vi "Read Operator Joystick.vi"   [LabVIEW 2020]
uses:
  Framework/Robot Global Data.vi
  <vilib>/Rock Robotics/Network Tables/NT Write Numeric Array.vi
  <vilib>/Rock Robotics/Network Tables/NT Write Boolean Array.vi
types:
  T1 = enum16{"0", "1", "2", "3", "4", "5", "6", "7", "8", "9", "10", "11"}
  T2 = typedef "WPI_JoystickDevRef.ctl" = cluster{"Device":T3}
  T3 = typedef "WPI_JoystickDeviceEnum.ctl" = enum16{"USB 0", "USB 1", "USB 2", "USB 3", "USB 4", "USB 5"}
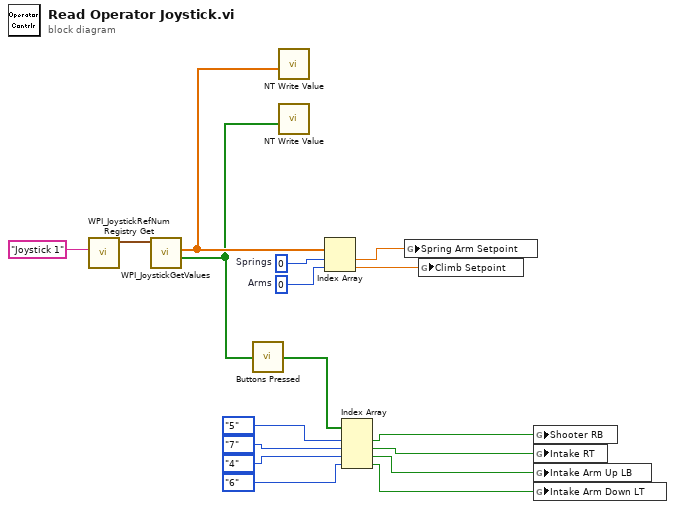
[diagram p0: block diagram]
diagram:
  w14 = 0  # Arms
  w15 = 0  # Springs
  n1 = call <vilib>:"WPI_JoystickRefNum Registry Get.vi"("refnum name"="Joystick 1") -> ("JoystickDevRef"=w17:T2)  [unwired: 9 in, 1 out]
  n2 = call <vilib>:"WPI_JoystickGetValues.vi"("JoystickDevRef"=w17) -> ("Buttons"=w12:bool[], "Axes"=w13:dbl[])  [unwired: 6 in, 3 out]
  n3 = call "Buttons Pressed.vi"("Button Values"=w12) -> ("Button Presses"=w11:bool[])
  n4 = call-poly <vilib>:"NT Write Value.vi"("Numeric Array"=w13) -> ()  [unwired: 10 in, 1 out]
  n5 = call-poly <vilib>:"NT Write Value.vi"("Boolean Array"=w12) -> ()  [unwired: 10 in, 1 out]
  n6 = Index Array(array=w13, index #1=w15, index #2=w14) -> (element #1=w10:dbl, element #2=w9:dbl)
  n7 = Index Array(array=w11, index #1=T1."5", index #2=T1."7", index #3=T1."4", index #4=T1."6") -> (element #1=w8:bool, element #2=w7:bool, element #3=w6:bool, element #4=w5:bool)
  n8 = global write "Robot Global Data.vi" "Spring Arm Setpoint"(w10) -> ()
  n9 = global write "Robot Global Data.vi" "Climb Setpoint"(w9) -> ()
  n10 = global write "Robot Global Data.vi" "Shooter RB"(w8) -> ()
  n11 = global write "Robot Global Data.vi" "Intake RT"(w7) -> ()
  n12 = global write "Robot Global Data.vi" "Intake Arm Up LB"(w6) -> ()
  n13 = global write "Robot Global Data.vi" "Intake Arm Down LT"(w5) -> ()
